vi "AddNextNode.vi"(6 "Variant in":variant, 7 "Shift Pressed?":bool, 8 "error in (no error)":errorcluster, 10 "QD Combo Box Ref":refnum<vi>, 11 "QD Launch VI Ref":refnum<vi>) -> (0 "error out":errorcluster, 4 "Variant out":variant)   [LabVIEW 2014]
doc: "Write a 1-2 sentence description of the functionality of your plugin here. Replace the \"$\" below with the character you wish to assign as the default shortcut for this plugin. Do not add any text after the 'Default Shortcut' line below.\n\nDefault Shortcut - [0]"
panel:
  in  "Undo Name":string="Quick Drop Keyboard Shortcut"
  # "Do not change the connector pane of this VI.\n\nSee the block diagram for directions on how to use this template."
  # "Specify the name of the Undo transaction"
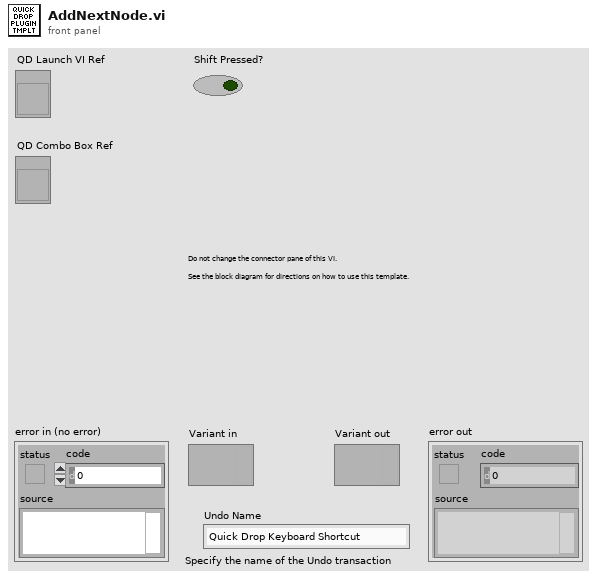
[diagram p1: front panel]
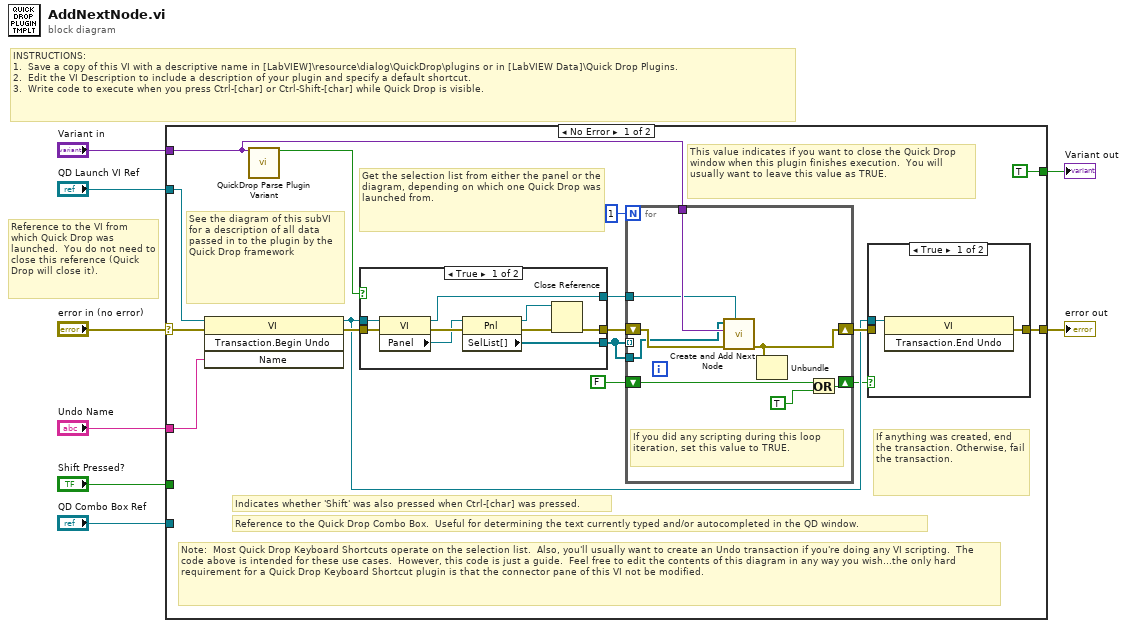
[diagram p0: block diagram]
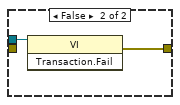
[diagram p2: hidden frame]
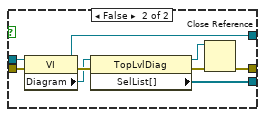
[diagram p3: hidden frame]
diagram:
  # "Reference to the VI from which Quick Drop was launched.  You do not need to close this reference (Quick Drop will close it)."
  # "INSTRUCTIONS:\n1.  Save a copy of this VI with a descriptive name in [LabVIEW]\\resource\\dialog\\QuickDrop\\plugins or in [LabVIEW Data]\\Quick Drop Plugins.\n2.  Edit the VI Description to include a description of your plugin and specify a default shortcut. \n3.  Write code to execute when you press Ctrl-[char] or Ctrl-Shift-[char] while Quick Drop is visible."
  n1 = case shown="No Error" "error in (no error)" {
    selector: "error in (no error)" -> [w24 w55]
    tunnel: [w18 w55] -> w7
    tunnel: "QD Launch VI Ref" -> [w23 _]
    tunnel: "Shift Pressed?" -> [_ _]
    tunnel: "QD Combo Box Ref" -> [_ _]
    tunnel: "Variant in" -> [w9 _]
    tunnel: "Undo Name" -> [w22 _]
    tunnel: [TRUE _] -> w1
    frame No Error {
      # "Note:  Most Quick Drop Keyboard Shortcuts operate on the selection list.  Also, you'll usually want to create an Undo transaction if you're doing any VI scripting.  The code above is intended for these use cases.  However, this code is just a guide.  Feel free to edit the contents of this diagram in any way you wish...the only hard requirement for a Quick Drop Keyboard Shortcut plugin is that the connector pane of this VI not be modified."
      # "Get the selection list from either the panel or the diagram, depending on which one Quick Drop was launched from."
      # "If anything was created, end the transaction. Otherwise, fail the transaction."
      # "This value indicates if you want to close the Quick Drop window when this plugin finishes execution.  You will usually want to leave this value as TRUE."
      # "See the diagram of this subVI for a description of all data passed in to the plugin by the Quick Drop framework"
      # "Reference to the Quick Drop Combo Box.  Useful for determining the text currently typed and/or autocompleted in the QD window."
      # "Indicates whether 'Shift' was also pressed when Ctrl-[char] was pressed."
      n2 = invoke class="VI" method="Transaction.Begin Undo"(reference=w23, error in=w24, "Name"=w22) -> (reference out=w15:refnum<vi>, error out=w19:errorcluster)  [unwired: 1 in, 2 out]
      n3 = call <vilib>:"QuickDrop Parse Plugin Variant.vi"("QDKS Variant in"=w9) -> ("QD Launch VI Panel?"=w20:bool)  [unwired: 12 in, 2 out]
      n4 = case shown="True" w20 {
        tunnel: w19 -> [w45 w54]
        tunnel: w15 -> [w44 w53]
        tunnel: [w39 w48] -> w17
        tunnel: [w38 w47] -> w11
        tunnel: [w37 w46] -> w10
        frame True {
          n5 = property class="VI"(reference=w44, error in=w45) -> (reference out=w37:refnum<vi>, error out=w43:errorcluster, "Panel"=w42:refnum<vi>)
          n6 = property class="Pnl"(reference=w42, error in=w43) -> (reference out=w40:refnum<vi>, error out=w41:errorcluster, "SelList[]"=w38:refnum<vi>[])
          n7 = Close Reference(reference=w40, error in (no error)=w41) -> (error out=w39:errorcluster)
        }
        frame False {
          n8 = property class="VI"(reference=w53, error in=w54) -> (reference out=w46:refnum<vi>, error out=w52:errorcluster, "Diagram"=w51:refnum<vi>)
          n9 = property class="TopLvlDiag"(reference=w51, error in=w52) -> (reference out=w49:refnum<vi>, error out=w50:errorcluster, "SelList[]"=w47:refnum<vi>[])
          n10 = Close Reference(reference=w49, error in (no error)=w50) -> (error out=w48:errorcluster)
        }
      }
      n11 = for {
        N: 1 -> [_]
        shift-right: [w27] -> w16
        shift-left: w17 -> [w30]
        shift-right: [w31] -> w13
        shift-left: FALSE -> [w32]
        tunnel: w11 -> [_] mode=indexing
        tunnel: w11 -> [w28]
        tunnel: w10 -> [w25]
        tunnel: w9 -> [w29]
        # "If you did any scripting during this loop iteration, set this value to TRUE."
        n12 = call <resource>:"Create and Add Next Node.vi"("VI Ref"=w25, "error in (no error)"=w30, "Variant in"=w29, "SelList[]"=w28) -> ("error out"=w27:errorcluster)  [unwired: 7 in]
        n13 = Unbundle(w27) -> ()  [unwired: 3 out]
        n14 = Or(x=w32, y=TRUE ("x")) -> (x .or. y?=w31:bool)
      }
      n15 = case shown="True" w13 {
        tunnel: w15 -> [w33 w35]
        tunnel: [w34 w36] -> w18
        tunnel: w16 -> [_ _]
        frame True {
          n16 = invoke class="VI" method="Transaction.End Undo"(reference=w33) -> (error out=w34:errorcluster)  [unwired: 2 in, 2 out]
        }
        frame False {
          n17 = invoke class="VI" method="Transaction.Fail"(reference=w35) -> (error out=w36:errorcluster)  [unwired: 2 in, 2 out]
        }
      }
    }
    frame Error {
    }
  }
  "error out" <- w7
  "Variant out" <- w1
